vi "niFpgaFifoEmulationRefIn.vi"(0 "Element in":variant, 1 "Method":T2, 2 "Input Valid":bool, 3 "Name":variant, 4 "Timeout":i32, 5 "error in (no error)":errorcluster, 6 "Type":variant, 7 "Width":i32, 8 "Ready for Output":bool, 11 "Node Link":cluster{"VIRef":refnum<vi>, "UID":i32}, 12 "In SCTL":bool) -> (13 "Ready for Input?":bool, 14 "Element out":variant, 15 "FullEmpty":bool, 16 "Output Valid":bool, 17 "Count":u32, 18 "StreamState":T1, 19 "error out":errorcluster)   [LabVIEW 2017]
uses:
  <vilib>/rvi/DataTransferAndStorage/Container/Common/niFpgaContainerMethod.ctl
  <vilib>/rvi/DataTransferAndStorage/FIFO/niFpgaPeerToPeerStreamState.ctl
  <vilib>/rvi/FIFO/Fifo_Types/niFpgaFifoControlLogicControl.ctl
  <vilib>/rvi/DataTransferAndStorage/Container/Common/niFpgaContainerMetaDataKey.ctl
  <instcachedir>/0/nirvififoEmulationWrite_A649243FB3B24943A09B1DA8A757A569.lvgen/nirvififoEmulationWrite_A649243FB3B24943A09B1DA8A757A569_000.vi
  <instcachedir>/0/nirvififoEmulationRead_3DFC15695E2B4FC5A392C1228151C501.lvgen/nirvififoEmulationRead_3DFC15695E2B4FC5A392C1228151C501_000.vi
  <instcachedir>/0/nirvififoEmulationClear_BF77B075DD414432B9FC23BE5F06EC6F.lvgen/nirvififoEmulationClear_BF77B075DD414432B9FC23BE5F06EC6F_000.vi
  <instcachedir>/0/nirvififoEmulationGetNumberOfElementsToRead_E57A145D2C234A4DAFE358F8BBE33451.lvgen/nirvififoEmulationGetNumberOfElementsToRead_E57A145D2C234A4DAFE358F8BBE33451_000.vi
  <instcachedir>/0/nirvififoEmulationGetNumberOfElementsToWrite_ADC517B29DC6482A80F74CD91CD1C0B3.lvgen/nirvififoEmulationGetNumberOfElementsToWrite_ADC517B29DC6482A80F74CD91CD1C0B3_000.vi
  <instcachedir>/0/nirviRandomDataFpgaReadWriteTemplate_4D4AFC2E39EF4A1ABFAEB8367EECF91C.lvgen/nirviRandomDataFpgaReadWriteTemplate_4D4AFC2E39EF4A1ABFAEB8367EECF91C_000.vi
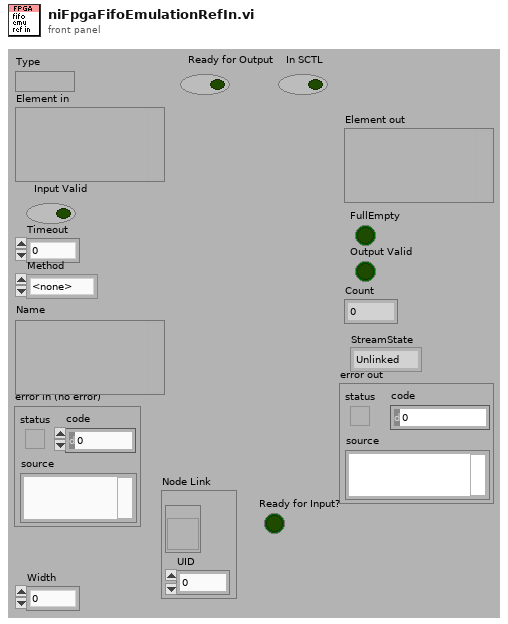
[diagram p1: front panel]
types:
  T1 = typedef "niFpgaPeerToPeerStreamState.ctl" = enum16{"Unlinked", "Disabled", "Enabled", "Flushing"}
  T2 = typedef "niFpgaContainerMethod.ctl" = enum16{"<none>", "write", "read", "clear", "getNumberOfElementsToWrite", "getNumberOfElementsToRead", "enable", "disable", "flushAndDisable", "getStreamState", "readA", "readB", "dramWrite", "dramWriteWithByteEnables", "dramRequestData", "dramRetrieveData", "readWithoutAcknowledge", "acknowledge", "writeUsingHandshaking", "readUsingHandshaking", "flush"}
  T3 = typedef "niFpgaFifoControlLogicControl.ctl" = enum16{"Slice Fabric", "Target Optimal", "Built-in"}
  T4 = typedef "niFpgaContainerMetaDataKey.ctl" = enum16{"FPGA FIFO", "FPGA Memory", "FPGA Register", "FPGA Handshake"}
  T5 = typedef "niFpgaContainerState.ctl" = cluster{"displayName":string, "hardwareName":string, "dataType":T6, "elementTypeDescriptor":variant, "terminalTypeDescriptor":variant, "requestedNumberOfElements":u32, "memoryType":T7, "arbitrationForInterfaceA":T8, "numberOfElementsPerRead":u32, "arbitrationForInterfaceB":T8, "numberOfElementsPerWrite":u32, "VI_Defined":bool, "type":T9, "initializationParameters":T10, "disableOnOverflow/Underflow":bool, "interfaceConfiguration":T11, "controlLogic":T3, "actualNumberOfElements":u32, "dramSelection":string, "dramMaxOustandingRequests":i32, "dramIncludeByteEnables":bool, "dramGrantTime":u32, "fullEmulation":bool, "memoryInMultipleClockDomains":bool, "memoryLatency":T12}
  T6 = typedef "niFpgaDataTypeControl.ctl" = enum32{"Boolean", "I8", "I16", "I32", "I64", "U8", "U16", "U32", "U64", "FXP", "CustomControl", "SGL"}
  T7 = typedef "niFpgaContainerImplementationControl.ctl" = enum16{"Flip-Flops", "Look-Up Table", "Block Memory", "DRAM"}
  T8 = typedef "niFpgaContainerArbitrationOptionsControl.ctl" = enum16{"Always Arbitrate", "Arbitrate if Multiple Requestors Only", "Never Arbitrate"}
  T9 = typedef "niFpgaTransferTypeControl.ctl" = enum16{"Target-Scoped", "Host to Target - DMA", "Target to Host - DMA", "Peer to Peer Reader", "Peer to Peer Writer", "Bidirectional"}
  T10 = typedef "niFpgaContainerInitializationParameters.ctl" = cluster{"initialized":bool, "VI_Path":path, "initialData":variant}
  T11 = typedef "niFpgaMemoryInterfaceConfiguration.ctl" = enum16{"Read A-Write B", "Read A-Read B"}
  T12 = typedef "niFpgaContainerMemoryLatencyControl.ctl" = u16
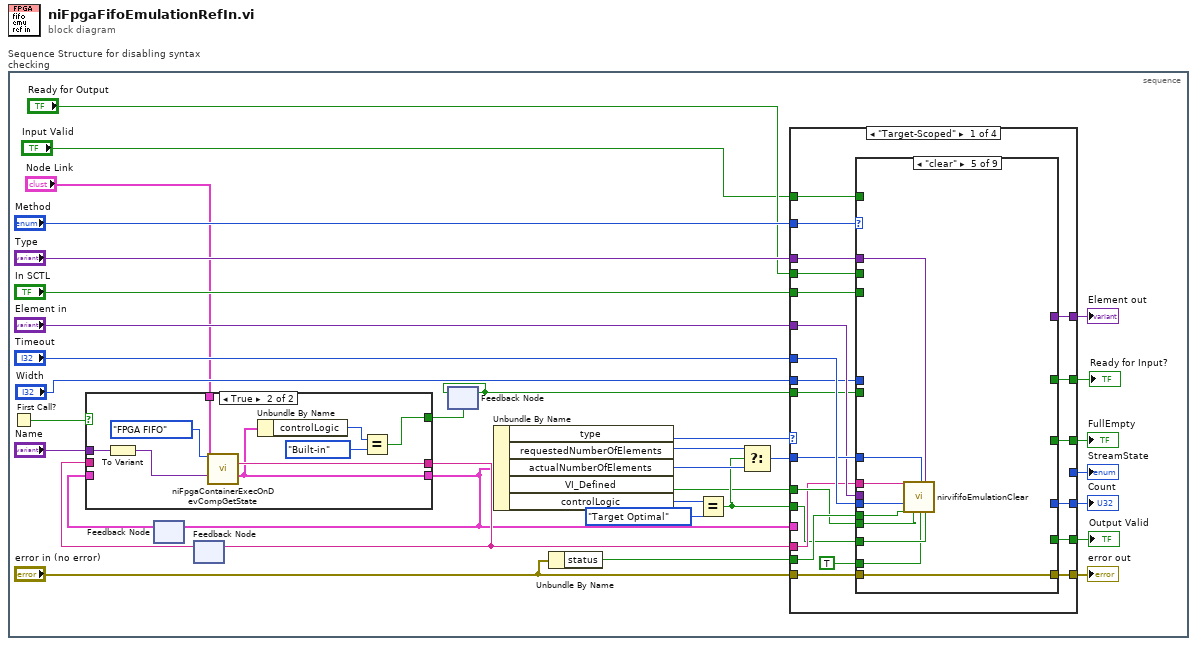
[diagram p0: block diagram]
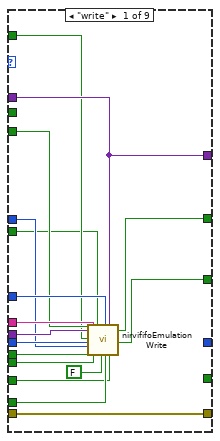
[diagram p2: hidden frame]
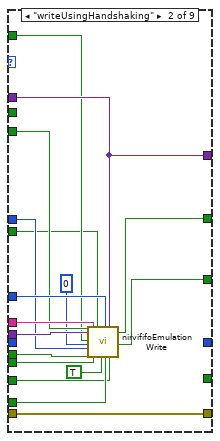
[diagram p3: hidden frame]
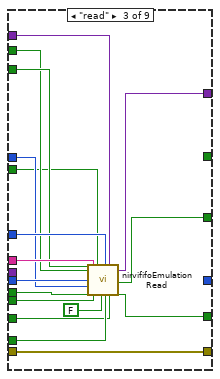
[diagram p4: hidden frame]
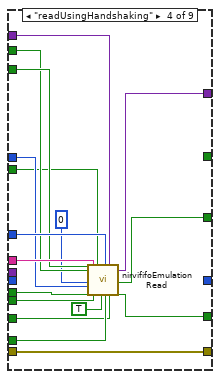
[diagram p5: hidden frame]
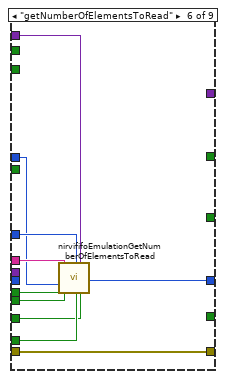
[diagram p6: hidden frame]
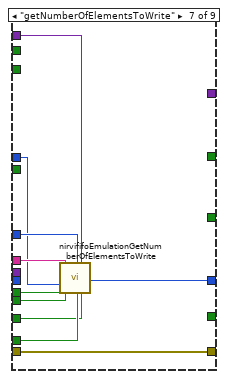
[diagram p7: hidden frame]
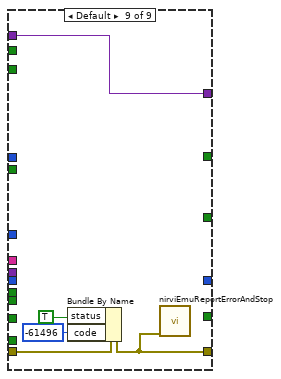
[diagram p9: hidden frame]
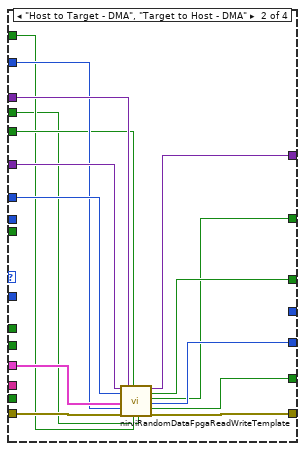
[diagram p10: hidden frame]
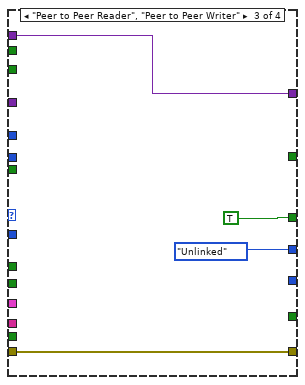
[diagram p11: hidden frame]
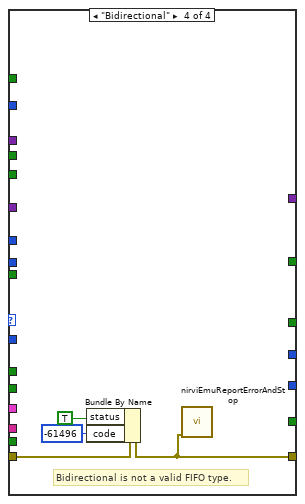
[diagram p12: hidden frame]
diagram:
  n1 = stacked-sequence "Sequence Structure for disabling syntax checking" {
    frame #0 {
      n2 = First Call?() -> (First Call?: T/F=w15:bool)
      n3 = feedback #1() -> (w18:T5)  [unwired: 1 out]
      n4 = feedback #2() -> (w25:string)  [unwired: 1 out]
      n5 = case shown="True" w15 {
        tunnel: [w184 w188] -> w24
        tunnel: w18 -> [w184 _]
        tunnel: "Name" -> [_ w193]
        tunnel: [w183 w192] -> w26
        tunnel: w25 -> [w183 _]
        tunnel: "Node Link" -> [_ w189]
        tunnel: [_ w185] -> w2
        frame False {
        }
        frame True {
          n6 = To Variant(anything=w193) -> (Variant=w190:variant)
          n7 = call <vilib>:"niFpgaContainerExecOnDevCompGetState.vi"("containerMetaDataKey"=niFpgaContainerMetaDataKey."FPGA FIFO", "Node Link"=w189, "name"=w190) -> ("Unique  Name"=w192:string, "containerState"=w188:T5)  [unwired: 3 in, 8 out]
          n8 = Unbundle By Name(w188) -> ("controlLogic"=w187:T3)
          n9 = Equal?(x=w187, y=niFpgaFifoControlLogicControl."Built-in") -> (x = y?=w185:bool)
        }
      }
      n10 = feedback-in #1(w24) -> ()
      n11 = feedback-in #2(w26) -> ()
      n12 = feedback #3(w2) -> (w1:bool)
      n13 = feedback-in #3(w1) -> ()
      n14 = Unbundle By Name(w24) -> ("type"=w23:T9, "requestedNumberOfElements"=w32:u32, "actualNumberOfElements"=w33:u32, "VI_Defined"=w17:bool, "controlLogic"=w28:T3)
      n15 = Unbundle By Name("error in (no error)") -> ("status"=w16:bool)
      n16 = Equal?(x=w28, y=niFpgaFifoControlLogicControl."Target Optimal") -> (x = y?=w31:bool)
      n17 = Select(t=w32, s=w31, f=w33) -> (s? t:f=w34:u32)
      n18 = case shown="\"Target-Scoped\"" w23 {
        tunnel: w16 -> [w56 _ _ _]
        tunnel: "Timeout" -> [w55 w171 _ _]
        tunnel: w34 -> [w54 _ _ _]
        tunnel: w17 -> [w53 _ _ _]
        tunnel: "Type" -> [w52 w169 w178 _]
        tunnel: [w51 w168 w178 _] -> w12
        tunnel: [w50 w167 TRUE ("Timed out") _] -> w10
        tunnel: "error in (no error)" -> [w49 w174 w177 w180]
        tunnel: [w48 w173 w177 w179] -> w11
        tunnel: "Method" -> [w47 w165 _ _]
        tunnel: "Element in" -> [w46 w170 _ _]
        tunnel: w24 -> [_ w172 _ _]
        tunnel: [w45 w166 _ _] -> w19
        tunnel: w26 -> [w44 _ _ _]
        tunnel: [_ _ niFpgaPeerToPeerStreamState."Unlinked" ("Stream State") _] -> w27
        tunnel: w31 -> [w42 _ _ _]
        tunnel: "Width" -> [w41 _ _ _]
        tunnel: "In SCTL" -> [w40 w164 _ _]
        tunnel: [w39 w162 _ _] -> w6
        tunnel: "Ready for Output" -> [w38 w160 _ _]
        tunnel: "Input Valid" -> [w37 w161 _ _]
        tunnel: [w36 w163 _ _] -> w3
        tunnel: w1 -> [w35 _ _ _]
        frame "Target-Scoped" {
          n19 = case shown="\"clear\"" w47 {
            tunnel: w56 -> [w72 w89 w107 w124 w126 w143 w153 _ _]
            tunnel: w55 -> [w70 _ w106 _ w132 _ _ _ _]
            tunnel: w54 -> [w68 w86 w105 w123 w125 w139 w149 _ _]
            tunnel: w44 -> [w69 w87 w104 w122 w131 w138 w148 _ _]
            tunnel: w53 -> [w71 w88 w103 w121 w127 w142 w152 _ _]
            tunnel: w52 -> [w65 w83 w102 w120 w130 w141 w151 _ w159]
            tunnel: [w65 w83 w101 w119 _ _ _ _ w159] -> w51
            tunnel: [w67 w85 w100 w118 _ _ _ _ _] -> w50
            tunnel: w49 -> [w66 w84 w99 w117 w133 w140 w150 w154 w156]
            tunnel: [w66 w84 w99 w117 w133 w140 w150 w154 w155] -> w48
            tunnel: w46 -> [w73 w90 _ _ _ _ _ _ _]
            tunnel: [_ _ _ _ _ w137 w147 _ _] -> w45
            tunnel: TRUE -> [w64 w82 w98 w116 w128 w136 w146 _ _]
            tunnel: w42 -> [w63 w81 w97 w115 w129 w135 w145 _ _]
            tunnel: w41 -> [w62 w80 w92 w114 _ w134 w144 _ _]
            tunnel: w40 -> [w61 w79 w96 w113 _ _ _ _ _]
            tunnel: [_ _ w95 w112 _ _ _ _ _] -> w39
            tunnel: w38 -> [_ _ w94 w111 _ _ _ _ _]
            tunnel: w37 -> [w60 w78 _ _ _ _ _ _ _]
            tunnel: [w59 w77 _ _ _ _ _ _ _] -> w36
            tunnel: w35 -> [w57 w74 w91 w108 _ _ _ _ _]
            frame "write" {
              n20 = call-generic <vilib>:"nirvififoEmulationWrite.vi"("In SCTL"=w61, "Element"=w73, "Input Valid"=w60, "Timeout"=w70, "Width"=w62, "ErrorIn"=w72, "Name"=w69, "Local? (F)"=w71, "Is Built-In FIFO?"=w57, "Is Handshake?"=FALSE, "Size"=w68, "ref in wired"=w64, "Type"=w65, "Update Size?"=w63) -> ("Ready for Input"=w59:bool, "Full"=w67:bool)  [unwired: 12 in]
            }
            frame "writeUsingHandshaking" {
              n21 = call-generic <vilib>:"nirvififoEmulationWrite.vi"("In SCTL"=w79, "Element"=w90, "Input Valid"=w78, "Timeout"=0, "Width"=w80, "ErrorIn"=w89, "Name"=w87, "Local? (F)"=w88, "Is Built-In FIFO?"=w74, "Is Handshake?"=TRUE, "Size"=w86, "ref in wired"=w82, "Type"=w83, "Update Size?"=w81) -> ("Ready for Input"=w77:bool, "Full"=w85:bool)  [unwired: 12 in]
            }
            frame "read" {
              n22 = call-generic <vilib>:"nirvififoEmulationRead.vi"("In SCTL"=w96, "Ready for Output"=w94, "Timeout"=w106, "Width"=w92, "ErrorIn"=w107, "Name"=w104, "Local? (F)"=w103, "Is Built-In FIFO?"=w91, "Is Handshake?"=FALSE, "Size"=w105, "ref in wired"=w98, "Type"=w102, "Update Size?"=w97) -> ("Element"=w101:variant, "Empty"=w100:bool, "Output Valid"=w95:bool)  [unwired: 12 in]
            }
            frame "readUsingHandshaking" {
              n23 = call-generic <vilib>:"nirvififoEmulationRead.vi"("In SCTL"=w113, "Ready for Output"=w111, "Timeout"=0, "Width"=w114, "ErrorIn"=w124, "Name"=w122, "Local? (F)"=w121, "Is Built-In FIFO?"=w108, "Is Handshake?"=TRUE, "Size"=w123, "ref in wired"=w116, "Type"=w120, "Update Size?"=w115) -> ("Element"=w119:variant, "Empty"=w118:bool, "Output Valid"=w112:bool)  [unwired: 12 in]
            }
            frame "clear" {
              n24 = call-generic <vilib>:"nirvififoEmulationClear.vi"("Width"=w132, "ErrorIn"=w126, "Name"=w131, "Local? (F)"=w127, "Size"=w125, "ref in wired"=w128, "Type"=w130, "Update Size?"=w129) -> ()  [unwired: 20 in]
            }
            frame "getNumberOfElementsToRead" {
              n25 = call-generic <vilib>:"nirvififoEmulationGetNumberOfElementsToRead.vi"("Width"=w134, "ErrorIn"=w143, "Name"=w138, "Local? (F)"=w142, "Size"=w139, "ref in wired"=w136, "Type"=w141, "Update Size?"=w135) -> ("Number of Elements to Read"=w137:i32)  [unwired: 19 in]
            }
            frame "getNumberOfElementsToWrite" {
              n26 = call-generic <vilib>:"nirvififoEmulationGetNumberOfElementsToWrite.vi"("Width"=w144, "ErrorIn"=w153, "Name"=w148, "Local? (F)"=w152, "Size"=w149, "ref in wired"=w146, "Type"=w151, "Update Size?"=w145) -> ("Number of Elements to Write"=w147:u32)  [unwired: 19 in]
            }
            frame "enable".."getStreamState" {
            }
            frame Default {
              n27 = Bundle By Name(cluster=w156, "status"=TRUE, "code"=-61496) -> (w155:errorcluster)
              n28 = call <vilib>:"nirviEmuReportErrorAndStop.vi"("error to report"=w155) -> ()  [unwired: 3 in, 12 out]
            }
          }
        }
        frame "Host to Target - DMA", "Target to Host - DMA" {
          n29 = call-generic <vilib>:"nirviRandomDataFpgaReadWriteTemplate.vi"("Element in"=w170, "Timeout (ms)"=w171, "Fifo"=w172, "Method"=w165, "error in (no error)"=w174, "type"=w169, "In SCTL"=w164, "Input Valid?"=w161, "Ready for Output?"=w160) -> ("element"=w168:variant, "Timed out"=w167:bool, "Ready for Input"=w163:bool, "count"=w166:u32, "Output Valid"=w162:bool, "error out"=w173:errorcluster)  [unwired: 5 in]
        }
        frame "Peer to Peer Reader", "Peer to Peer Writer" {
        }
        frame "Bidirectional" {
          # "Bidirectional is not a valid FIFO type."
          n30 = Bundle By Name(cluster=w180, "status"=TRUE, "code"=-61496) -> (w179:errorcluster)
          n31 = call <vilib>:"nirviEmuReportErrorAndStop.vi"("error to report"=w179) -> ()  [unwired: 3 in, 12 out]
        }
      }
      "FullEmpty" <- w10
      "error out" <- w11
      "Element out" <- w12
      "Count" <- w19
      "StreamState" <- w27
      "Output Valid" <- w6
      "Ready for Input?" <- w3
    }
  }
